vi "Calibrate Current.vi"(8 "error in (no error)":errorcluster, 10 "Current (A)":dbl, 11 "Reload-pro in":refnum<class "Reload-pro.lvclass">) -> (0 "error out":errorcluster, 3 "Reload-pro out":refnum<class "Reload-pro.lvclass">)   [LabVIEW 2013, in "Reload-pro.lvclass"]
uses:
  Reload-pro.lvclass
panel:
  out "Response":string
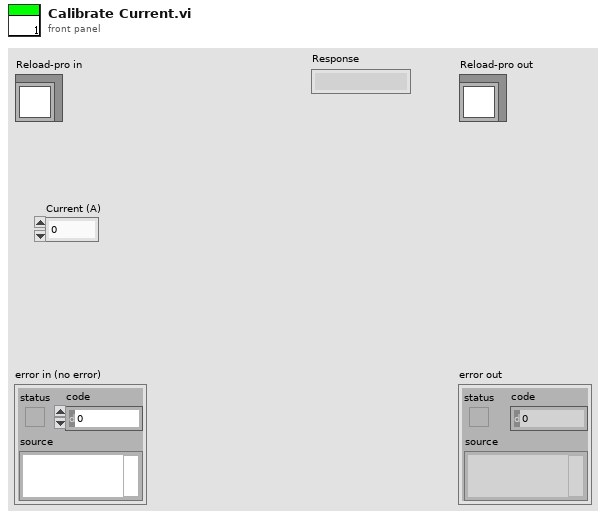
[diagram p1: front panel]
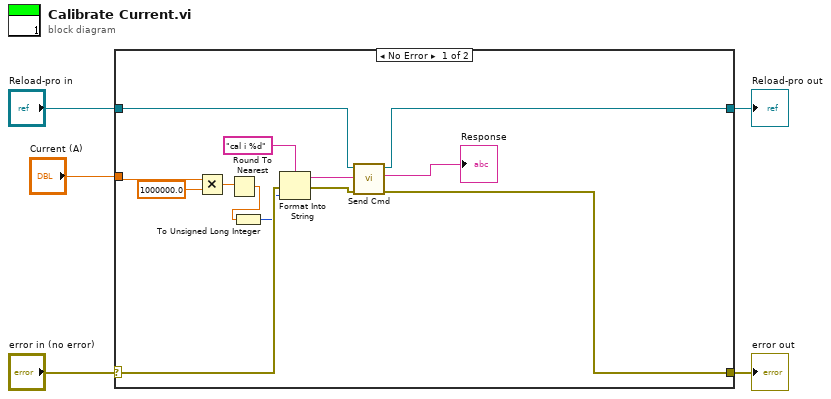
[diagram p0: block diagram]
diagram:
  n1 = case shown="No Error" "error in (no error)" {
    selector: "error in (no error)" -> [w12 w20]
    tunnel: [w11 w20] -> w4
    tunnel: [w9 w19] -> w2
    tunnel: "Reload-pro in" -> [w10 w19]
    tunnel: "Current (A)" -> [w18 _]
    frame No Error {
      n2 = Multiply(x=w18, y=1000000.0) -> (x*y=w16:dbl)
      n3 = Round To Nearest(number=w16) -> (nearest integer value=w7:dbl)
      n4 = To Unsigned Long Integer(number=w7) -> (unsigned 32bit integer=w6:u32)
      n5 = Format Into String(format string="cal i %d", error in=w12, w6) -> (resulting string=w14:string, error out=w13:errorcluster)  [unwired: 1 in]
      n6 = call-dynamic "Send Cmd.vi"("error in (no error)"=w13, "Command"=w14, "Reload-pro in"=w10) -> ("error out"=w11:errorcluster, "Response"=→"Response":string, "Reload-pro out"=w9:refnum<class "Reload-pro.lvclass">)  [unwired: 6 in]
    }
    frame Error {
    }
  }
  "error out" <- w4
  "Reload-pro out" <- w2
